vi "RamCtrl_SimDiffDrive_Exec.vi"(8 "error in (no error)":errorcluster) -> (0 "error out":errorcluster, 1 "Left Motor Vel - PV (Ft/Sec)":dbl format="%20.3f", 2 "Right Motor Dist (Ft)":dbl format="%20.3f", 3 "Left Motor Dist (Ft)":dbl format="%20.3f", 4 "Gyro Heading (Deg)":dbl format="%20.3f", 5 "Left Motor Dmd":dbl format="%20.3f", 6 "Right Motor Vel - PV (Ft/Sec)":dbl format="%20.3f", 7 "Right Motor Dmd":dbl format="%20.3f")   [LabVIEW 2019]
uses:
  <vilib>/Rock Robotics/WPI/ThirdParty/JAS_Junk/TrajLib/Enum/DIFF_DRIVE_TRAIN_SIM_STATE_ENUM.ctl
  <vilib>/Rock Robotics/WPI/ThirdParty/JAS_Junk/TrajLib/Enum/DIFF_DRIVE_KitBot_WheelSize_ENUM.ctl
  <vilib>/Rock Robotics/WPI/ThirdParty/JAS_Junk/TrajLib/Enum/DIFF_DRIVE_ToughBoxMini_GearChoice_ENUM.ctl
  <vilib>/Rock Robotics/WPI/ThirdParty/JAS_Junk/TrajLib/Enum/DCMOTOR_TYPES_ENUM.ctl
  <vilib>/Rock Robotics/WPI/ThirdParty/JAS_Junk/TrajLib/BatterySim_CalculateLoadedBatteryVoltage.vi
  <vilib>/Rock Robotics/WPI/ThirdParty/JAS_Junk/TrajLib/Units_InchesToMeters.vi
  <vilib>/Rock Robotics/WPI/ThirdParty/JAS_Junk/TrajLib/VI/numCmd_ObtainQueue_TwoDbl.vi
  <vilib>/Rock Robotics/WPI/ThirdParty/JAS_Junk/TrajLib/VI/numCmd_ObtainQueue_Array.vi
  <vilib>/Rock Robotics/WPI/ThirdParty/JAS_Junk/TrajLib/Conv_Inches_Meters.vi
  <vilib>/Rock Robotics/WPI/ThirdParty/JAS_Junk/TrajLib/Trajectory_Library.lvlib
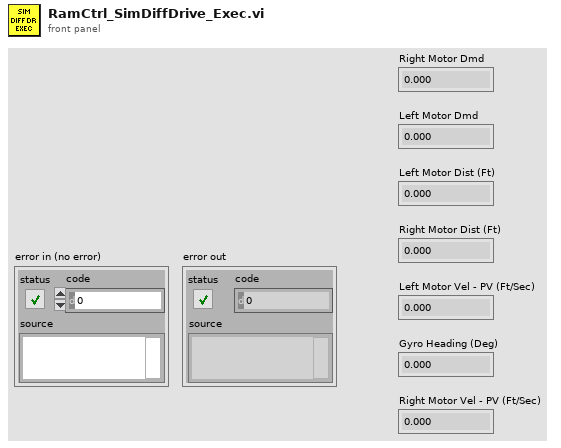
[diagram p1: front panel]
types:
  T1 = typedef "Trajectory_Library.lvlib/DIFF_DRIVE_TRAIN_SIM_STATE_ENUM.ctl" = enum16{"X_POS", "Y_POS", "HEADING", "LEFT_VEL", "RIGHT_VEL", "LEFT_DIST", "RIGHT_DIST"}
  T2 = typedef "Trajectory_Library.lvlib/DIFF_DRIVE_KitBot_WheelSize_ENUM.ctl" = enum16{"4 Inch", "6 Inch", "8 Inch", "10 Inch"}
  T3 = typedef "Trajectory_Library.lvlib/DIFF_DRIVE_ToughBoxMini_GearChoice_ENUM.ctl" = enum16{"Ratio_12_75", "Ratio_10_71", "Ratio_8_45", "Ratio_7_31", "Ratio_5_95"}
  T4 = typedef "Trajectory_Library.lvlib/DCMOTOR_TYPES_ENUM.ctl" = enum16{"CIM", "AndyMark 9015", "Andy Mark RS 775 125", "Bag", "BaneBots RS 550", "BaneBots RS 775", "Falcon 500", "Mini CIM", "NEO", "NEO 550", "Romi BuiltIn", "Vex 775 Pro", "Snow Blower AM 2235A", "Bosch Seat AM 3493"}
  T5 = typedef "Trajectory_Library.lvlib/DIFF_DRIVE_SIM_SIMULATION_PARAMS.ctl" = cluster{"X Pos Meas Std Dev M":dbl, "Y Pos Meas Std Dev M":dbl, "Heading Meas Std Dev Rad":dbl, "Left Vel Meas Std Dev M/S":dbl, "Right Vel Meas Std Dev M/S":dbl, "Left Pos Meas Std Dev M":dbl, "Right Pos Meas Std Dev M":dbl}
  T6 = typedef "Trajectory_Library.lvlib/DIFF_DRIVE_SIM_MODEL_PARAMS.CTL" = cluster{"TracWidth_M":dbl, "WheelRadius_M":dbl, "Gearing":dbl, "Mass kg":dbl, "MOI kgm2":dbl, "DCMOTOR_TYPES":T4, "Num Motors":i32}
  T7 = typedef "Trajectory_Library.lvlib/DIFF_DRIVE_TRAIN_SIM.ctl" = cluster{"m_Plant":T8, "m_X":T9, "m_Y":T9, "m_U":T9, "MeasureStdDev":T9, "m_Motor":T10, "m_OriginalGearing":dbl, "m_CurrentGearing":dbl, "m_WheelRadius_M":dbl, "m_RB":dbl}
  T8 = typedef "Trajectory_Library.lvlib/LINEAR_SYSTEM.ctl" = cluster{"m_A":T9, "m_B":T9, "m_C":T9, "m_D":T9, "States":i32, "Inputs":i32, "Outputs":i32}
  T9 = typedef "NI_Matrix.lvlib/RealMatrix.ctl" = dbl[][]
  T10 = typedef "Trajectory_Library.lvlib/DCMOTOR.CTL" = cluster{"nominalVoltage_Volts":dbl, "StallTorque_NM":dbl, "StallCurrent_Amps":dbl, "FreeCurrent_Amps":dbl, "FreeSpeed_RadPerSec":dbl, "R_Ohms":dbl, "KvINV_RadPerSecPerVolt":dbl, "Kt_NMPerAmp":dbl, "L_H":dbl, "Jr_KgM2":dbl}
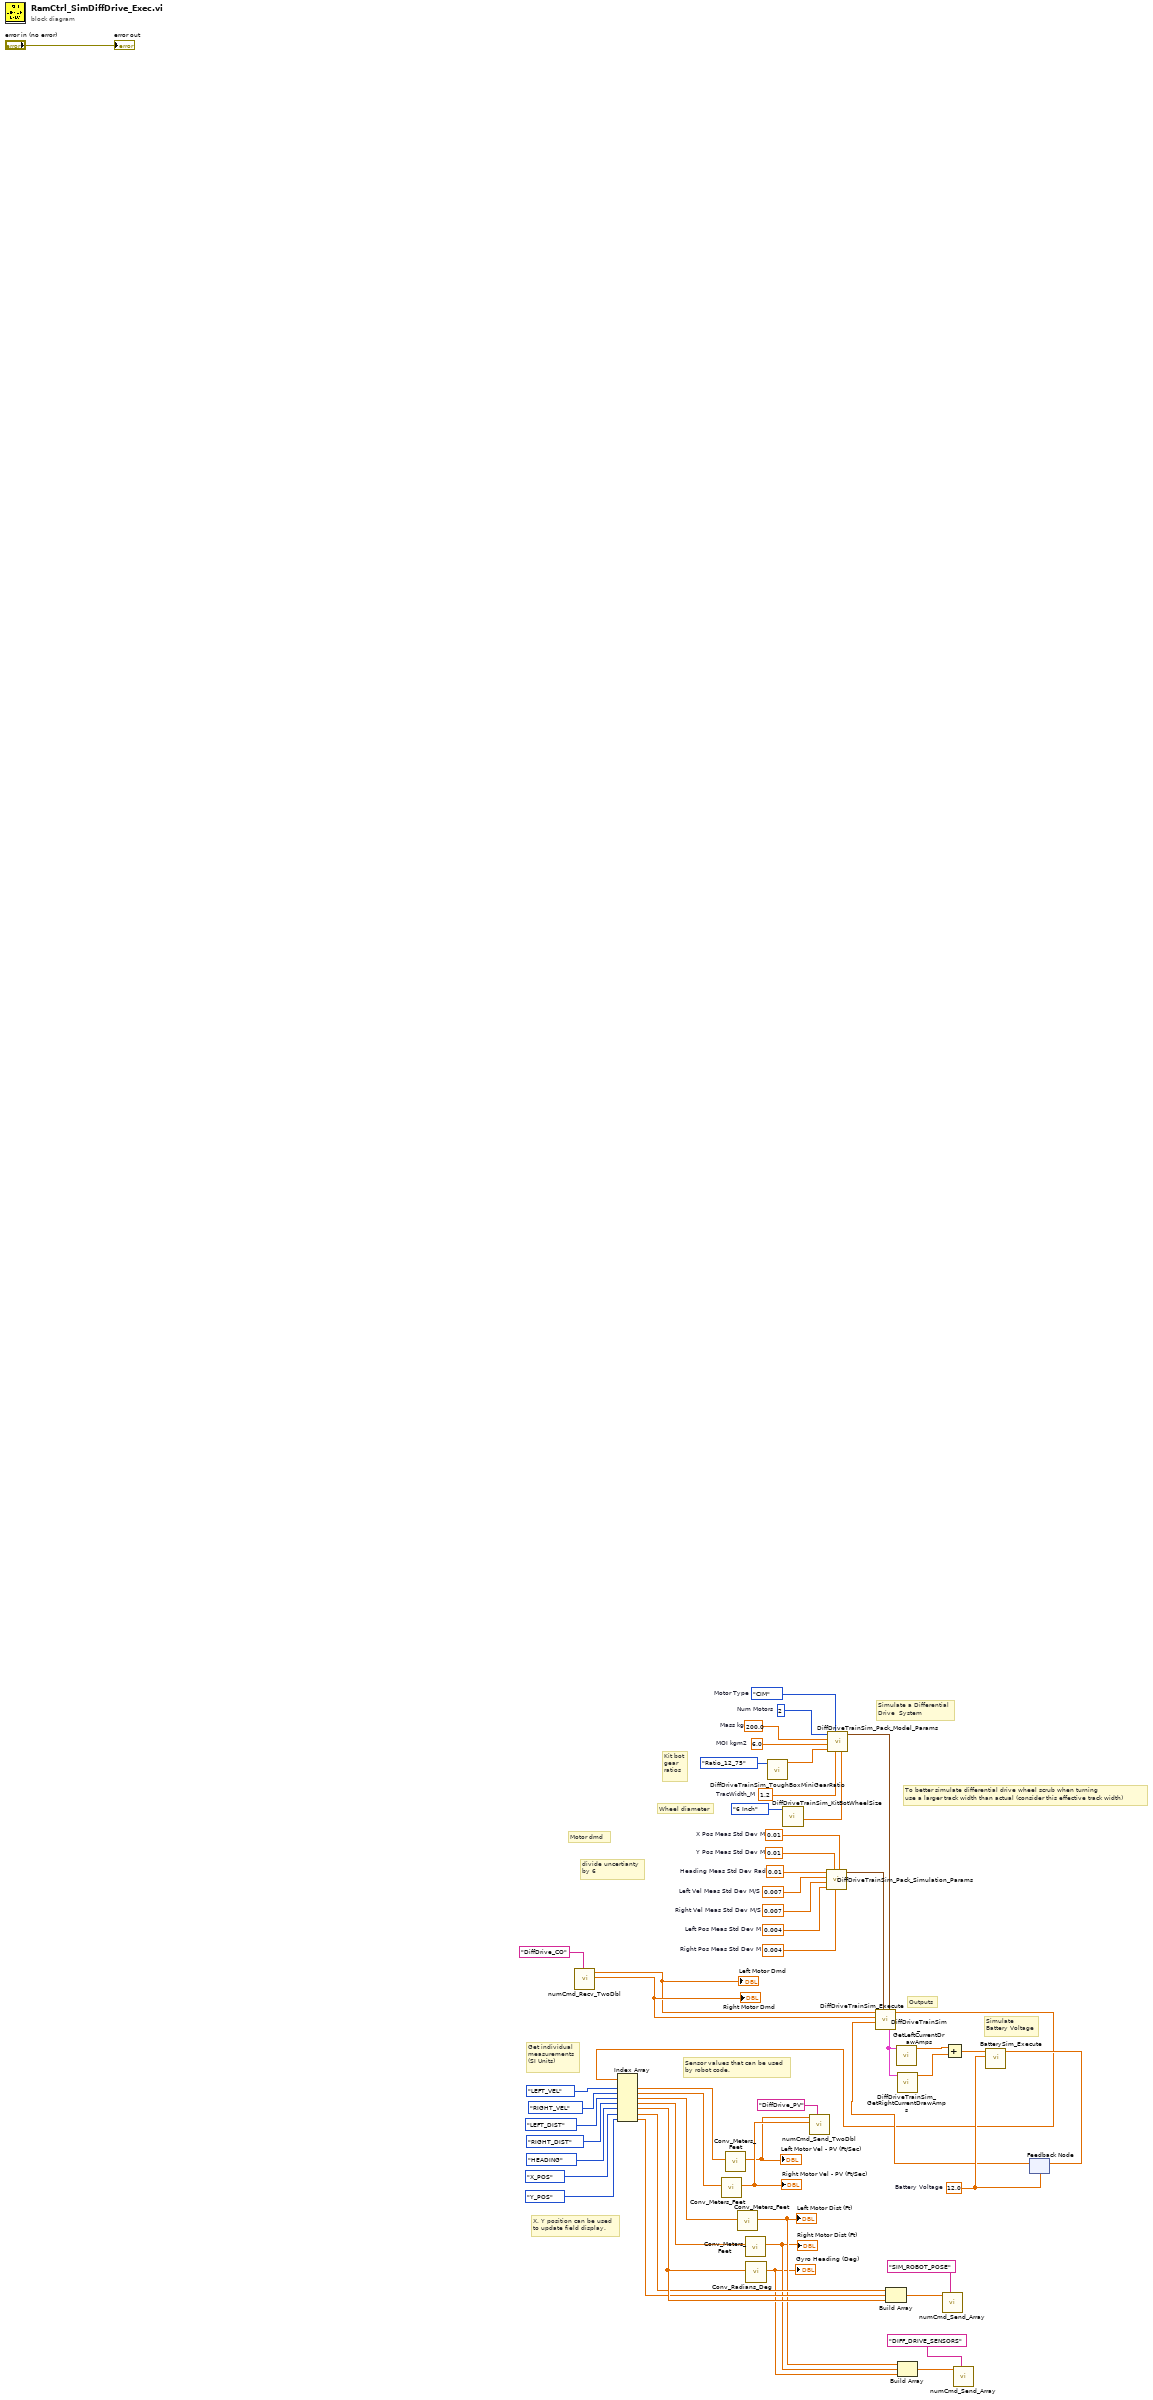
[diagram p0: block diagram]
diagram:
  w54 = 12.0  # Battery Voltage
  w20 = 200.0  # Mass kg
  w19 = 6.0  # MOI kgm2
  w18 = 1.2  # TracWidth_M
  w17 = 0.01  # Heading Meas Std Dev Rad
  w16 = 0.007  # Left Vel Meas Std Dev M/S
  w15 = 0.007  # Right Vel Meas Std Dev M/S
  w14 = 0.004  # Left Pos Meas Std Dev M
  w13 = 0.01  # Y Pos Meas Std Dev M
  w12 = 0.004  # Right Pos Meas Std Dev M
  w11 = 0.01  # X Pos Meas Std Dev M
  w8 = 2  # Num Motors
  w7 = DCMOTOR_TYPES_ENUM."CIM"  # Motor Type
  # "divide uncertianty\nby 6"
  # "To better simulate differential drive wheel scrub when turning\nuse a larger track width than actual (consider this effective track width)"
  # "Sensor values that can be used\nby robot code."
  # "X, Y position can be used\nto update field display."
  # "Motor dmd"
  # "Wheel diameter"
  # "Get individual\nmeasurements\n(SI Units)"
  # "Kit bot\ngear \nratios"
  # "Outputs"
  # "Simulate\nBattery Voltage"
  # "Simulate a Differential\nDrive  System"
  n1 = call <vilib>:"numCmd_Recv_TwoDbl.vi"("Command Name"="DiffDrive_CO") -> ("Value 2"=w45:dbl, "Value 1"=w44:dbl)  [unwired: 7 in, 2 out]
  "Left Motor Dmd" <- w44
  "Right Motor Dmd" <- w45
  n2 = call <vilib>:"DiffDriveTrainSim_ToughBoxMiniGearRatio.vi"("ToughBoxMiniGear"=DIFF_DRIVE_ToughBoxMini_GearChoice_ENUM."Ratio_12_75") -> ("GearRatio"=w22:dbl)  [unwired: 10 in]
  n3 = call <vilib>:"DiffDriveTrainSim_KitBotWheelSize.vi"("Wheel Size"=DIFF_DRIVE_KitBot_WheelSize_ENUM."6 Inch") -> ("WheelRadius_M"=w30:dbl)  [unwired: 9 in, 1 out]
  n4 = call <vilib>:"DiffDriveTrainSim_Pack_Simulation_Params.vi"("X Pos Meas Std Dev M"=w11, "Right Pos Meas Std Dev M"=w12, "Y Pos Meas Std Dev M"=w13, "Left Pos Meas Std Dev M"=w14, "Right Vel Meas Std Dev M/S"=w15, "Left Vel Meas Std Dev M/S"=w16, "Heading Meas Std Dev Rad"=w17) -> ("DiffDriveSim_Simulation _Params"=w10:T5)  [unwired: 4 in]
  n5 = call <vilib>:"DiffDriveTrainSim_Pack_Model_Params.vi"("WheelRadius_M"=w30, "TracWidth_M"=w18, "DCMOTOR_TYPES"=w7, "Gearing"=w22, "MOI kgm2"=w19, "Mass kg"=w20, "Num Motors"=w8) -> ("DiffDriveSim_Model _Params"=w9:T6)  [unwired: 4 in]
  n6 = feedback #1(w54) -> (w53:dbl)
  n7 = call <vilib>:"DiffDriveTrainSim_Execute.vi"("LinearSystem_ID_DiffDrv_Model"=w9, "DiffDriveSim_Simulation _Params"=w10, "BatteryVoltage"=w53, "Right Motor Dmd"=w45, "Left Motor Dmd"=w44) -> ("Outputs"=w51:dbl[], "out DiffDriveTrainSim"=w31:T7)  [unwired: 4 in, 1 out]
  n8 = Index Array(array=w51, index #1=DIFF_DRIVE_TRAIN_SIM_STATE_ENUM."LEFT_VEL" ("DIFF_DRIVE_TRAIN_SIM_STATE"), index #2=DIFF_DRIVE_TRAIN_SIM_STATE_ENUM."RIGHT_VEL" ("DIFF_DRIVE_TRAIN_SIM_STATE"), index #3=DIFF_DRIVE_TRAIN_SIM_STATE_ENUM."LEFT_DIST" ("DIFF_DRIVE_TRAIN_SIM_STATE"), index #4=DIFF_DRIVE_TRAIN_SIM_STATE_ENUM."RIGHT_DIST" ("DIFF_DRIVE_TRAIN_SIM_STATE"), index #5=DIFF_DRIVE_TRAIN_SIM_STATE_ENUM."HEADING" ("DIFF_DRIVE_TRAIN_SIM_STATE"), index #6=DIFF_DRIVE_TRAIN_SIM_STATE_ENUM."X_POS" ("DIFF_DRIVE_TRAIN_SIM_STATE"), index #7=DIFF_DRIVE_TRAIN_SIM_STATE_ENUM."Y_POS" ("DIFF_DRIVE_TRAIN_SIM_STATE")) -> (element #1=w32:dbl, element #2=w33:dbl, element #3=w34:dbl, element #4=w35:dbl, element #5=w48:dbl, element #6=w46:dbl, element #7=w47:dbl)
  n9 = call <vilib>:"Conv_Meters_Feet.vi"("Meters"=w33) -> ("Feet"=w43:dbl)  [unwired: 10 in]
  "Right Motor Vel - PV (Ft/Sec)" <- w43
  n10 = call <vilib>:"Conv_Meters_Feet.vi"("Meters"=w32) -> ("Feet"=w42:dbl)  [unwired: 10 in]
  "Left Motor Vel - PV (Ft/Sec)" <- w42
  n11 = call <vilib>:"Conv_Meters_Feet.vi"("Meters"=w34) -> ("Feet"=w3:dbl)  [unwired: 10 in]
  "Left Motor Dist (Ft)" <- w3
  n12 = call <vilib>:"Conv_Meters_Feet.vi"("Meters"=w35) -> ("Feet"=w2:dbl)  [unwired: 10 in]
  "Right Motor Dist (Ft)" <- w2
  n13 = call <vilib>:"Conv_Radians_Deg.vi"("Radians"=w48) -> ("Degrees"=w1:dbl)  [unwired: 10 in]
  "Gyro Heading (Deg)" <- w1
  n14 = call <vilib>:"numCmd_Send_TwoDbl.vi"("Command Name"="DiffDrive_PV", "Value 2"=w43, "Value 1"=w42) -> ()  [unwired: 8 in, 1 out]
  n15 = Build Array(w46, w47, w48) -> (w50:dbl[])
  n16 = call <vilib>:"DiffDriveTrainSim_GetLeftCurrentDrawAmps.vi"("DiffDriveTrainSim"=w31) -> ("LeftCurrentDraw_Amps"=w36:dbl)  [unwired: 10 in]
  n17 = call <vilib>:"DiffDriveTrainSim_GetRightCurrentDrawAmps.vi"("DiffDriveTrainSim"=w31) -> ("RightCurrentDraw_Amps"=w37:dbl)  [unwired: 10 in]
  n18 = Build Array(w3, w2, w1) -> (w5:dbl[])
  n19 = call <vilib>:"numCmd_Send_Array.vi"("Command Name"="SIM_ROBOT_POSE", "Values"=w50) -> ()  [unwired: 9 in, 1 out]
  n20 = Add(x=w36, y=w37) -> (x+y=w23:dbl)
  n21 = call <vilib>:"numCmd_Send_Array.vi"("Command Name"="DIFF_DRIVE_SENSORS", "Values"=w5) -> ()  [unwired: 9 in, 1 out]
  n22 = call <vilib>:"BatterySim_Execute.vi"("Nominal Battery Voltage"=w54, "Current"=w23) -> ("Voltage"=w52:dbl)  [unwired: 9 in]
  n23 = feedback-in #1(w52) -> ()
  "error out" <- "error in (no error)"
